vi "CAN Get CAL data.vi"(8 "error in":errorcluster, 11 "file (use dialog)":path) -> (0 "error out":errorcluster, 3 "CAL Data Bytes":u8[](array[numeric]) format="%.0x")   [LabVIEW 2014]
panel:
  in  "input string":string
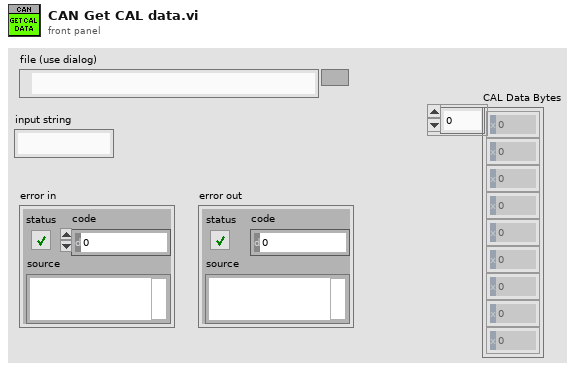
[diagram p1: front panel]
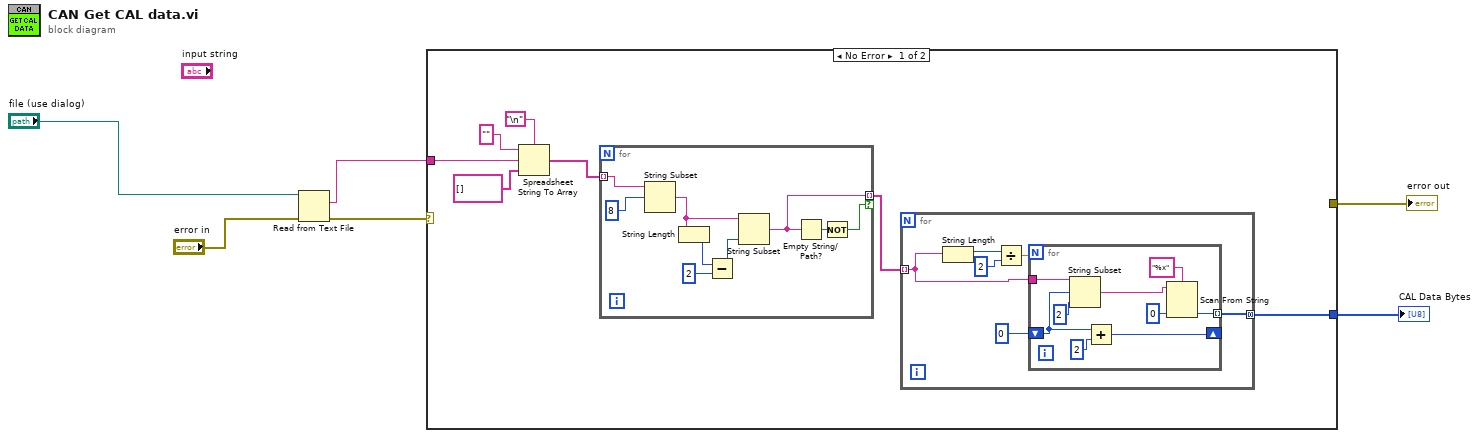
[diagram p0: block diagram]
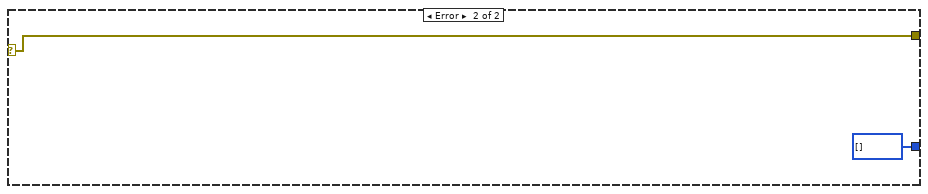
[diagram p2: hidden frame]
diagram:
  n1 = Read from Text File(file (use dialog)="file (use dialog)", error in="error in") -> (text=w1:string, error out=w5:errorcluster)  [unwired: 2 in, 2 out]
  n2 = case shown="No Error" w5 {
    selector: w5 -> [_ w38]
    tunnel: w1 -> [w13 _]
    tunnel: [w7 u8[] []] -> w3
    tunnel: [_ w38] -> w2
    frame No Error {
      n3 = Spreadsheet String To Array(delimiter (Tab)="\n", format string="", spreadsheet string=w13, array type (2D Dbl)=string[] [] ("Array")) -> (array=w9:string[])
      n4 = for {
        tunnel: w9 -> [w37] mode=indexing
        tunnel: [w29] -> w8 mode=indexing if=w30
        n5 = String Subset(string=w37, offset (0)=8) -> (substring=w32:string)  [unwired: 1 in]
        n6 = String Length(string=w32) -> (length=w35:i32)
        n7 = Subtract(x=w35, y=2) -> (x-y=w33:i32)
        n8 = String Subset(string=w32, length (rest)=w33) -> (substring=w29:string)  [unwired: 1 in]
        n9 = Empty String/Path?(string/path=w29) -> (empty?=w31:bool)
        n10 = Not(x=w31) -> (.not. x?=w30:bool)
      }
      n11 = for {
        tunnel: w8 -> [w14] mode=indexing
        tunnel: [w15] -> w7 mode=concatenating
        n12 = String Length(string=w14) -> (length=w18:i32)
        n13 = Divide(x=w18, y=2) -> (x/y=w16:dbl)
        n14 = for {
          N: w16 -> [_]
          tunnel: w14 -> [w28]
          shift-right: [w26] -> _
          shift-left: 0 -> [w24]
          tunnel: [w20] -> w15 mode=indexing
          n15 = String Subset(string=w28, offset (0)=w24, length (rest)=2 ("length (rest)")) -> (substring=w21:string)
          n16 = Add(x=w24, y=2) -> (x+y=w26:i32)
          n17 = Scan From String(format string="%x", input string=w21, default 1=u8 0 ("default value 1")) -> (output 1=w20:u8)  [unwired: 2 in, 3 out]
        }
      }
    }
    frame Error {
    }
  }
  "error out" <- w2
  "CAL Data Bytes" <- w3
